vi "modbus slave new.vi"() -> ()   [LabVIEW 2016, in "MB SLAVE.lvlib"]
uses:
  MB SLAVE.lvlib
  <vilib>/NI/Modbus Library/Network Protocol/Network Slave/daemon status.ctl
  <vilib>/NI/Modbus Library/Network Protocol/Network Slave/TCP/Connection.ctl
  <vilib>/NI/Modbus Library/API/Wrapper/Create TCP Slave.vi
  <vilib>/NI/Modbus Library/API/slave/Modbus Slave.lvclass
  <vilib>/NI/Modbus Library/API/Wrapper/API Main.lvlib
  <vilib>/ptbypt/NI_PtbyPt.lvlib
  <vilib>/NI/Modbus Library/Network Protocol/Network Slave/Network Slave.lvclass
  <vilib>/NI/Modbus Library/Network Protocol/Network Slave/TCP/TCP Slave.lvclass
panel:
  in  "写入采配水关键参数":u16[](array[numeric])
  in  "写入校准点信息":u16[](array[numeric])
  in  "写入关键参数":u16[](array[numeric])
  in  "写入各参数测量间隔":u16[](array[numeric])
  out "读取各参数测量间隔":u16[](array[numeric])
  in  "写入试剂余量":u16[](array[numeric])
  out "TCP Connection List":T1[](array[typedef])
  out "TCP Connection Count":u32
  out "Daemon Status":T2
  out "读取关键参数":u16[](array[numeric])
  out "status":bool
  in  "写入系统仪器状态":u16[](array[numeric])
  out "读取反控命令":u16[](array[numeric])
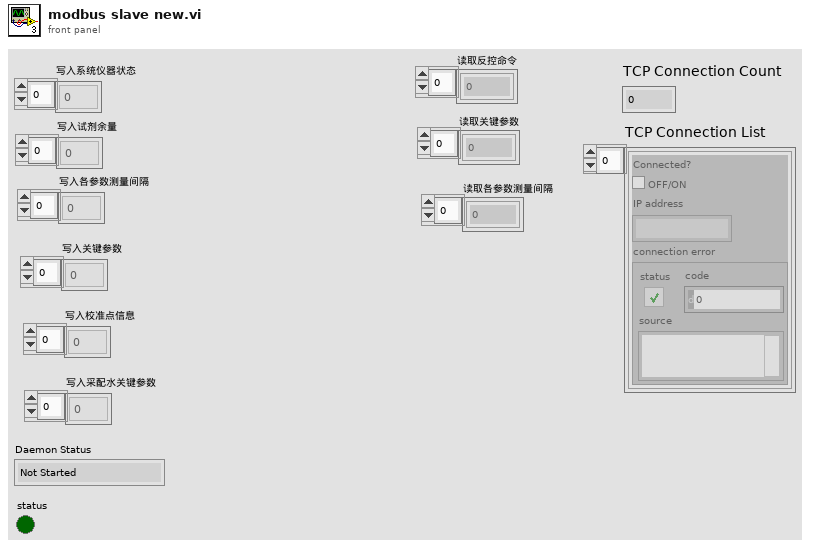
[diagram p1: front panel]
types:
  T1 = typedef "TCP Slave.lvclass/Connection.ctl" = cluster{"Connected?":bool, "IP address":string, "connection error":errorcluster}
  T2 = typedef "Network Slave.lvclass/daemon status.ctl" = enum16{"Not Started", "Running", "Error", "Stopped"}
  T3 = typedef "系统交互.ctl" = cluster{"运行模式":enum16{"维护模式", "常规模式", "应急模式", "质控模式", "性能测试"}, "运行间隔":i16, "流程运行中":bool, "自动运行启动参数":T4, "SYSTEM Interface.总磷总氮类型":enum16{"单模块", "总磷总氮二合一模块", "氨氮总磷二合一模块"}, "多参数运行间隔":i16, "配水时间":dbl, "沉淀时间":dbl, "清洗时间":dbl, "关键参数改变":bool, "温度告警":bool, "湿度告警":bool, "烟感告警":bool, "水浸告警":bool, "开门告警":bool, "SystemTask":enum16{"停机", "待机", "调试", "水样采集", "沉沙", "进样", "仪表测试分析", "反吹", "清洗", "除藻"}, "PumpState":enum16{"--", "只用泵1", "只用泵2", "双泵交替"}, "除藻选择":enum16{"不开除藻", "开除藻"}, "报警信息":enum16{"无报警", "断电报警", "采样管理欠压（源水泵故障）", "进样管路欠压（进样泵/增加泵故障）"}, "软件升级":bool}
  T4 = typedef "启动参数.ctl" = cluster{"氨氮":bool, "总磷":bool, "总氮":bool, "多参数":bool, "CODmn":bool, "CODCr":bool, "氟化物":bool, "超标留样":bool, "重金属":bool, "挥发酚":bool}
  T5 = typedef "多参数交互.ctl" = cluster{"pH":bool, "DO":bool, "Turb":bool, "Cond":bool, "Temp":bool, "叶绿素a启用":bool, "蓝绿藻":bool, "藻密度":bool, "orp":bool}
  T6 = typedef "CODMn交互.ctl" = cluster{"COD浓度（mg/L)":dbl, "水样启动时间":timestamp, "加标回收启动时间":timestamp, "CODMn工作状态":enum16{"空闲", "水样测试", "标样核查", "零点核查", "跨度核查", "空白测试", "平行样测试", "加标回收", "空白校准", "标样校准", "初始化（清洗）"}, "多列列表框":i32, "平台试剂余量百分比":sgl, "关键参数":cluster{"测量量程":dbl, "测量精度":dbl, "测量间隔":dbl, "消解温度":dbl, "消解时长":dbl, "空白校准时间":timestamp, "曲线截距":dbl, "曲线斜率":dbl, "测量检出限":dbl, "测量信号值":dbl, "线性相关系数":dbl, "二次多项式系数":dbl, "标样校准时间":timestamp, "稀释倍数":dbl, "三项式系数":dbl, "空白标定系数":dbl, "量程系数":dbl, "F0/ORPA":dbl, "F1/ORPB":dbl, "F2/ORPK":dbl, "F3":dbl, "F4":dbl, "F5":dbl, "F6":dbl, "F7":dbl, "X0/滴定数":dbl, "量程":dbl}, "关键参数改变":bool, "校准信息":cluster{"低标液1浓度":dbl, "低标液1信号值":dbl, "低标液1启用":u16, "低标液2浓度":dbl, "低标液2信号值":dbl, "低标液2启用":u16, "低标液3浓度":dbl, "低标液3信号值":dbl, "低标液3启用":u16, "低标液4浓度":dbl, "低标液4信号值":dbl, "低标液4启用":u16, "低标液5浓度":dbl, "低标液5信号值":dbl, "低标液5启用":u16, "高标液1浓度":dbl, "高标液1信号值":dbl, "高标液1启用":u16, "高标液2浓度":dbl, "高标液2信号值":dbl, "高标液2启用":u16, "高标液3浓度":dbl, "高标液3信号值":dbl, "高标液3启用":u16, "高标液4浓度":dbl, "高标液4信号值":dbl, "高标液4启用":u16, "高标液5浓度":dbl, "高标液5信号值":dbl, "高标液5启用":u16, "低斜率":dbl, "低截距":dbl, "低二次多项式系数":dbl, "低线性相关系数":dbl, "高斜率":dbl, "高截距":dbl, "高二次多项式系数":dbl, "高线性相关系数":dbl}, "校准信息改变":bool}
  T7 = typedef "CODCr交互.ctl" = cluster{"状态告警区":cluster{"系统时间":timestamp, "工作状态":u16, "测量模式":enum16{"待机", "连续模式", "周期模式", "定点模式", "受控模式", "手动模式"}, "告警代码":u16, "故障代码":u16, "日志代码":u16, "软件版本":u16, "F0":sgl, "F1":sgl, "F2":sgl, "F3":sgl, "T":sgl, "H":sgl, "id":u16, "flowid":u16, "量程":u16, "总磷控温温度1":sgl, "营养盐控温温度2":sgl, "ADC":sgl}, "平台试剂余量百分比":sgl, "关键参数":cluster{"测量量程":dbl, "测量精度":dbl, "测量间隔":dbl, "消解温度":dbl, "消解时长":dbl, "空白校准时间":timestamp, "曲线截距":dbl, "曲线斜率":dbl, "测量检出限":dbl, "测量信号值":dbl, "线性相关系数":dbl, "二次多项式系数":dbl, "标样校准时间":timestamp, "稀释倍数":dbl, "三项式系数":dbl, "空白标定系数":dbl, "量程系数":dbl, "F0/ORPA":dbl, "F1/ORPB":dbl, "F2/ORPK":dbl, "F3":dbl, "F4":dbl, "F5":dbl, "F6":dbl, "F7":dbl, "X0/滴定数":dbl, "量程":dbl}, "关键参数改变":bool, "校准信息":cluster{"低标液1浓度":dbl, "低标液1信号值":dbl, "低标液1启用":u16, "低标液2浓度":dbl, "低标液2信号值":dbl, "低标液2启用":u16, "低标液3浓度":dbl, "低标液3信号值":dbl, "低标液3启用":u16, "低标液4浓度":dbl, "低标液4信号值":dbl, "低标液4启用":u16, "低标液5浓度":dbl, "低标液5信号值":dbl, "低标液5启用":u16, "高标液1浓度":dbl, "高标液1信号值":dbl, "高标液1启用":u16, "高标液2浓度":dbl, "高标液2信号值":dbl, "高标液2启用":u16, "高标液3浓度":dbl, "高标液3信号值":dbl, "高标液3启用":u16, "高标液4浓度":dbl, "高标液4信号值":dbl, "高标液4启用":u16, "高标液5浓度":dbl, "高标液5信号值":dbl, "高标液5启用":u16, "低斜率":dbl, "低截距":dbl, "低二次多项式系数":dbl, "低线性相关系数":dbl, "高斜率":dbl, "高截距":dbl, "高二次多项式系数":dbl, "高线性相关系数":dbl}, "校准信息改变":bool}
  T8 = typedef "氨氮交互.ctl" = cluster{"状态告警区":cluster{"系统时间":timestamp, "工作状态":u16, "测量模式":enum16{"待机", "连续模式", "周期模式", "定点模式", "受控模式", "手动模式"}, "告警代码":u16, "故障代码":u16, "日志代码":u16, "软件版本":u16, "F0":sgl, "F1":sgl, "F2":sgl, "F3":sgl, "T":sgl, "H":sgl, "id":u16, "flowid":u16, "量程":u16, "总磷控温温度1":sgl, "营养盐控温温度2":sgl, "ADC":sgl}, "平台试剂余量百分比":sgl, "关键参数":cluster{"测量量程":dbl, "测量精度":dbl, "测量间隔":dbl, "消解温度":dbl, "消解时长":dbl, "空白校准时间":timestamp, "曲线截距":dbl, "曲线斜率":dbl, "测量检出限":dbl, "测量信号值":dbl, "线性相关系数":dbl, "二次多项式系数":dbl, "标样校准时间":timestamp, "稀释倍数":dbl, "三项式系数":dbl, "空白标定系数":dbl, "量程系数":dbl, "F0/ORPA":dbl, "F1/ORPB":dbl, "F2/ORPK":dbl, "F3":dbl, "F4":dbl, "F5":dbl, "F6":dbl, "F7":dbl, "X0/滴定数":dbl, "量程":dbl}, "关键参数改变":bool, "校准信息":cluster{"低标液1浓度":dbl, "低标液1信号值":dbl, "低标液1启用":u16, "低标液2浓度":dbl, "低标液2信号值":dbl, "低标液2启用":u16, "低标液3浓度":dbl, "低标液3信号值":dbl, "低标液3启用":u16, "低标液4浓度":dbl, "低标液4信号值":dbl, "低标液4启用":u16, "低标液5浓度":dbl, "低标液5信号值":dbl, "低标液5启用":u16, "高标液1浓度":dbl, "高标液1信号值":dbl, "高标液1启用":u16, "高标液2浓度":dbl, "高标液2信号值":dbl, "高标液2启用":u16, "高标液3浓度":dbl, "高标液3信号值":dbl, "高标液3启用":u16, "高标液4浓度":dbl, "高标液4信号值":dbl, "高标液4启用":u16, "高标液5浓度":dbl, "高标液5信号值":dbl, "高标液5启用":u16, "低斜率":dbl, "低截距":dbl, "低二次多项式系数":dbl, "低线性相关系数":dbl, "高斜率":dbl, "高截距":dbl, "高二次多项式系数":dbl, "高线性相关系数":dbl}, "校准信息改变":bool}
  T9 = typedef "总磷交互.ctl" = cluster{"状态告警区":cluster{"系统时间":timestamp, "工作状态":u16, "测量模式":enum16{"待机", "连续模式", "周期模式", "定点模式", "受控模式", "手动模式"}, "告警代码":u16, "故障代码":u16, "日志代码":u16, "软件版本":u16, "F0":sgl, "F1":sgl, "F2":sgl, "F3":sgl, "T":sgl, "H":sgl, "id":u16, "flowid":u16, "量程":u16, "总磷控温温度1":sgl, "营养盐控温温度2":sgl, "ADC":sgl}, "平台试剂余量百分比":sgl, "关键参数":cluster{"测量量程":dbl, "测量精度":dbl, "测量间隔":dbl, "消解温度":dbl, "消解时长":dbl, "空白校准时间":timestamp, "曲线截距":dbl, "曲线斜率":dbl, "测量检出限":dbl, "测量信号值":dbl, "线性相关系数":dbl, "二次多项式系数":dbl, "标样校准时间":timestamp, "稀释倍数":dbl, "三项式系数":dbl, "空白标定系数":dbl, "量程系数":dbl, "F0/ORPA":dbl, "F1/ORPB":dbl, "F2/ORPK":dbl, "F3":dbl, "F4":dbl, "F5":dbl, "F6":dbl, "F7":dbl, "X0/滴定数":dbl, "量程":dbl}, "关键参数改变":bool, "校准信息":cluster{"低标液1浓度":dbl, "低标液1信号值":dbl, "低标液1启用":u16, "低标液2浓度":dbl, "低标液2信号值":dbl, "低标液2启用":u16, "低标液3浓度":dbl, "低标液3信号值":dbl, "低标液3启用":u16, "低标液4浓度":dbl, "低标液4信号值":dbl, "低标液4启用":u16, "低标液5浓度":dbl, "低标液5信号值":dbl, "低标液5启用":u16, "高标液1浓度":dbl, "高标液1信号值":dbl, "高标液1启用":u16, "高标液2浓度":dbl, "高标液2信号值":dbl, "高标液2启用":u16, "高标液3浓度":dbl, "高标液3信号值":dbl, "高标液3启用":u16, "高标液4浓度":dbl, "高标液4信号值":dbl, "高标液4启用":u16, "高标液5浓度":dbl, "高标液5信号值":dbl, "高标液5启用":u16, "低斜率":dbl, "低截距":dbl, "低二次多项式系数":dbl, "低线性相关系数":dbl, "高斜率":dbl, "高截距":dbl, "高二次多项式系数":dbl, "高线性相关系数":dbl}, "校准信息改变":bool}
  T10 = typedef "总氮交互.ctl" = cluster{"状态告警区":cluster{"系统时间":timestamp, "工作状态":u16, "测量模式":enum16{"待机", "连续模式", "周期模式", "定点模式", "受控模式", "手动模式"}, "告警代码":u16, "故障代码":u16, "日志代码":u16, "软件版本":u16, "F0":sgl, "F1":sgl, "F2":sgl, "F3":sgl, "T":sgl, "H":sgl, "id":u16, "flowid":u16, "量程":u16, "总磷控温温度1":sgl, "营养盐控温温度2":sgl, "ADC":sgl}, "平台试剂余量百分比":sgl, "关键参数":cluster{"测量量程":dbl, "测量精度":dbl, "测量间隔":dbl, "消解温度":dbl, "消解时长":dbl, "空白校准时间":timestamp, "曲线截距":dbl, "曲线斜率":dbl, "测量检出限":dbl, "测量信号值":dbl, "线性相关系数":dbl, "二次多项式系数":dbl, "标样校准时间":timestamp, "稀释倍数":dbl, "三项式系数":dbl, "空白标定系数":dbl, "量程系数":dbl, "F0/ORPA":dbl, "F1/ORPB":dbl, "F2/ORPK":dbl, "F3":dbl, "F4":dbl, "F5":dbl, "F6":dbl, "F7":dbl, "X0/滴定数":dbl, "量程":dbl}, "关键参数改变":bool, "校准信息":cluster{"低标液1浓度":dbl, "低标液1信号值":dbl, "低标液1启用":u16, "低标液2浓度":dbl, "低标液2信号值":dbl, "低标液2启用":u16, "低标液3浓度":dbl, "低标液3信号值":dbl, "低标液3启用":u16, "低标液4浓度":dbl, "低标液4信号值":dbl, "低标液4启用":u16, "低标液5浓度":dbl, "低标液5信号值":dbl, "低标液5启用":u16, "高标液1浓度":dbl, "高标液1信号值":dbl, "高标液1启用":u16, "高标液2浓度":dbl, "高标液2信号值":dbl, "高标液2启用":u16, "高标液3浓度":dbl, "高标液3信号值":dbl, "高标液3启用":u16, "高标液4浓度":dbl, "高标液4信号值":dbl, "高标液4启用":u16, "高标液5浓度":dbl, "高标液5信号值":dbl, "高标液5启用":u16, "低斜率":dbl, "低截距":dbl, "低二次多项式系数":dbl, "低线性相关系数":dbl, "高斜率":dbl, "高截距":dbl, "高二次多项式系数":dbl, "高线性相关系数":dbl}, "校准信息改变":bool}
  T11 = cluster{"测量量程":dbl, "测量精度":dbl, "测量间隔":dbl, "消解温度":dbl, "消解时长":dbl, "空白校准时间":timestamp, "曲线截距":dbl, "曲线斜率":dbl, "测量检出限":dbl, "测量信号值":dbl, "线性相关系数":dbl, "二次多项式系数":dbl, "标样校准时间":timestamp, "稀释倍数":dbl, "三项式系数":dbl, "空白标定系数":dbl, "量程系数":dbl, "F0/ORPA":dbl, "F1/ORPB":dbl, "F2/ORPK":dbl, "F3":dbl, "F4":dbl, "F5":dbl, "F6":dbl, "F7":dbl, "X0/滴定数":dbl, "量程":dbl}
  T12 = cluster{"低标液1浓度":dbl, "低标液1信号值":dbl, "低标液1启用":u16, "低标液2浓度":dbl, "低标液2信号值":dbl, "低标液2启用":u16, "低标液3浓度":dbl, "低标液3信号值":dbl, "低标液3启用":u16, "低标液4浓度":dbl, "低标液4信号值":dbl, "低标液4启用":u16, "低标液5浓度":dbl, "低标液5信号值":dbl, "低标液5启用":u16, "高标液1浓度":dbl, "高标液1信号值":dbl, "高标液1启用":u16, "高标液2浓度":dbl, "高标液2信号值":dbl, "高标液2启用":u16, "高标液3浓度":dbl, "高标液3信号值":dbl, "高标液3启用":u16, "高标液4浓度":dbl, "高标液4信号值":dbl, "高标液4启用":u16, "高标液5浓度":dbl, "高标液5信号值":dbl, "高标液5启用":u16, "低斜率":dbl, "低截距":dbl, "低二次多项式系数":dbl, "低线性相关系数":dbl, "高斜率":dbl, "高截距":dbl, "高二次多项式系数":dbl, "高线性相关系数":dbl}
  T13 = enum16{"空闲", "水样测试", "标样核查", "零点核查", "跨度核查", "空白测试", "平行样测试", "加标回收", "空白校准", "标样校准", "初始化（清洗）"}
  T14 = typedef "超标留样交互.ctl" = cluster{"当前瓶号":u16}
  T15 = cluster{"测量量程":dbl, "测量精度":dbl, "测量间隔":dbl, "消解温度":dbl, "消解时长":dbl, "空白校准时间":timestamp, "曲线截距":dbl, "曲线斜率":dbl, "测量检出限":dbl, "测量信号值":dbl, "线性相关系数":dbl, "二次多项式系数":dbl, "标样校准时间":timestamp, "稀释倍数":dbl, "三项式系数":dbl, "空白标定系数":dbl, "量程系数":dbl, "F0/ORPA":dbl, "F1/ORPB":dbl, "F2/ORPK":dbl, "F3":dbl, "F4":dbl, "F5":dbl, "F6":dbl, "F7":dbl, "X0/滴定数":dbl, "量程":dbl}[]
  T16 = cluster{"低标液1浓度":dbl, "低标液1信号值":dbl, "低标液1启用":u16, "低标液2浓度":dbl, "低标液2信号值":dbl, "低标液2启用":u16, "低标液3浓度":dbl, "低标液3信号值":dbl, "低标液3启用":u16, "低标液4浓度":dbl, "低标液4信号值":dbl, "低标液4启用":u16, "低标液5浓度":dbl, "低标液5信号值":dbl, "低标液5启用":u16, "高标液1浓度":dbl, "高标液1信号值":dbl, "高标液1启用":u16, "高标液2浓度":dbl, "高标液2信号值":dbl, "高标液2启用":u16, "高标液3浓度":dbl, "高标液3信号值":dbl, "高标液3启用":u16, "高标液4浓度":dbl, "高标液4信号值":dbl, "高标液4启用":u16, "高标液5浓度":dbl, "高标液5信号值":dbl, "高标液5启用":u16, "低斜率":dbl, "低截距":dbl, "低二次多项式系数":dbl, "低线性相关系数":dbl, "高斜率":dbl, "高截距":dbl, "高二次多项式系数":dbl, "高线性相关系数":dbl}[]
  T17 = enum16{"启动整机", "停止整机", "标样核查", "加标回收", "平行样测试", "零点核查", "跨度核查", "校零", "校标"}
  T18 = cluster{"status":bool, "代码":u16, "source":string}
  T19 = enum16{"", "CODMn", "PH", "氨氮", "总氮", "总磷", "CODCr", "电导率", "水温", "溶解氧", "浊度", "叶绿素", "藻密度", "ORP"}
  T20 = enum16{"i13001", "i13002", "i13003", "i13004", "i13005", "i13006", "i13007", "i13008", "i13009", "i13010", "i13011", "i13012", "i13013", "i13014", "i13015", "i13016", "i13017", "i13101", "i13102", "i13103", "i13104", "i13105", "i13106", "i13107", "i13108", "i13109", "i13110"}
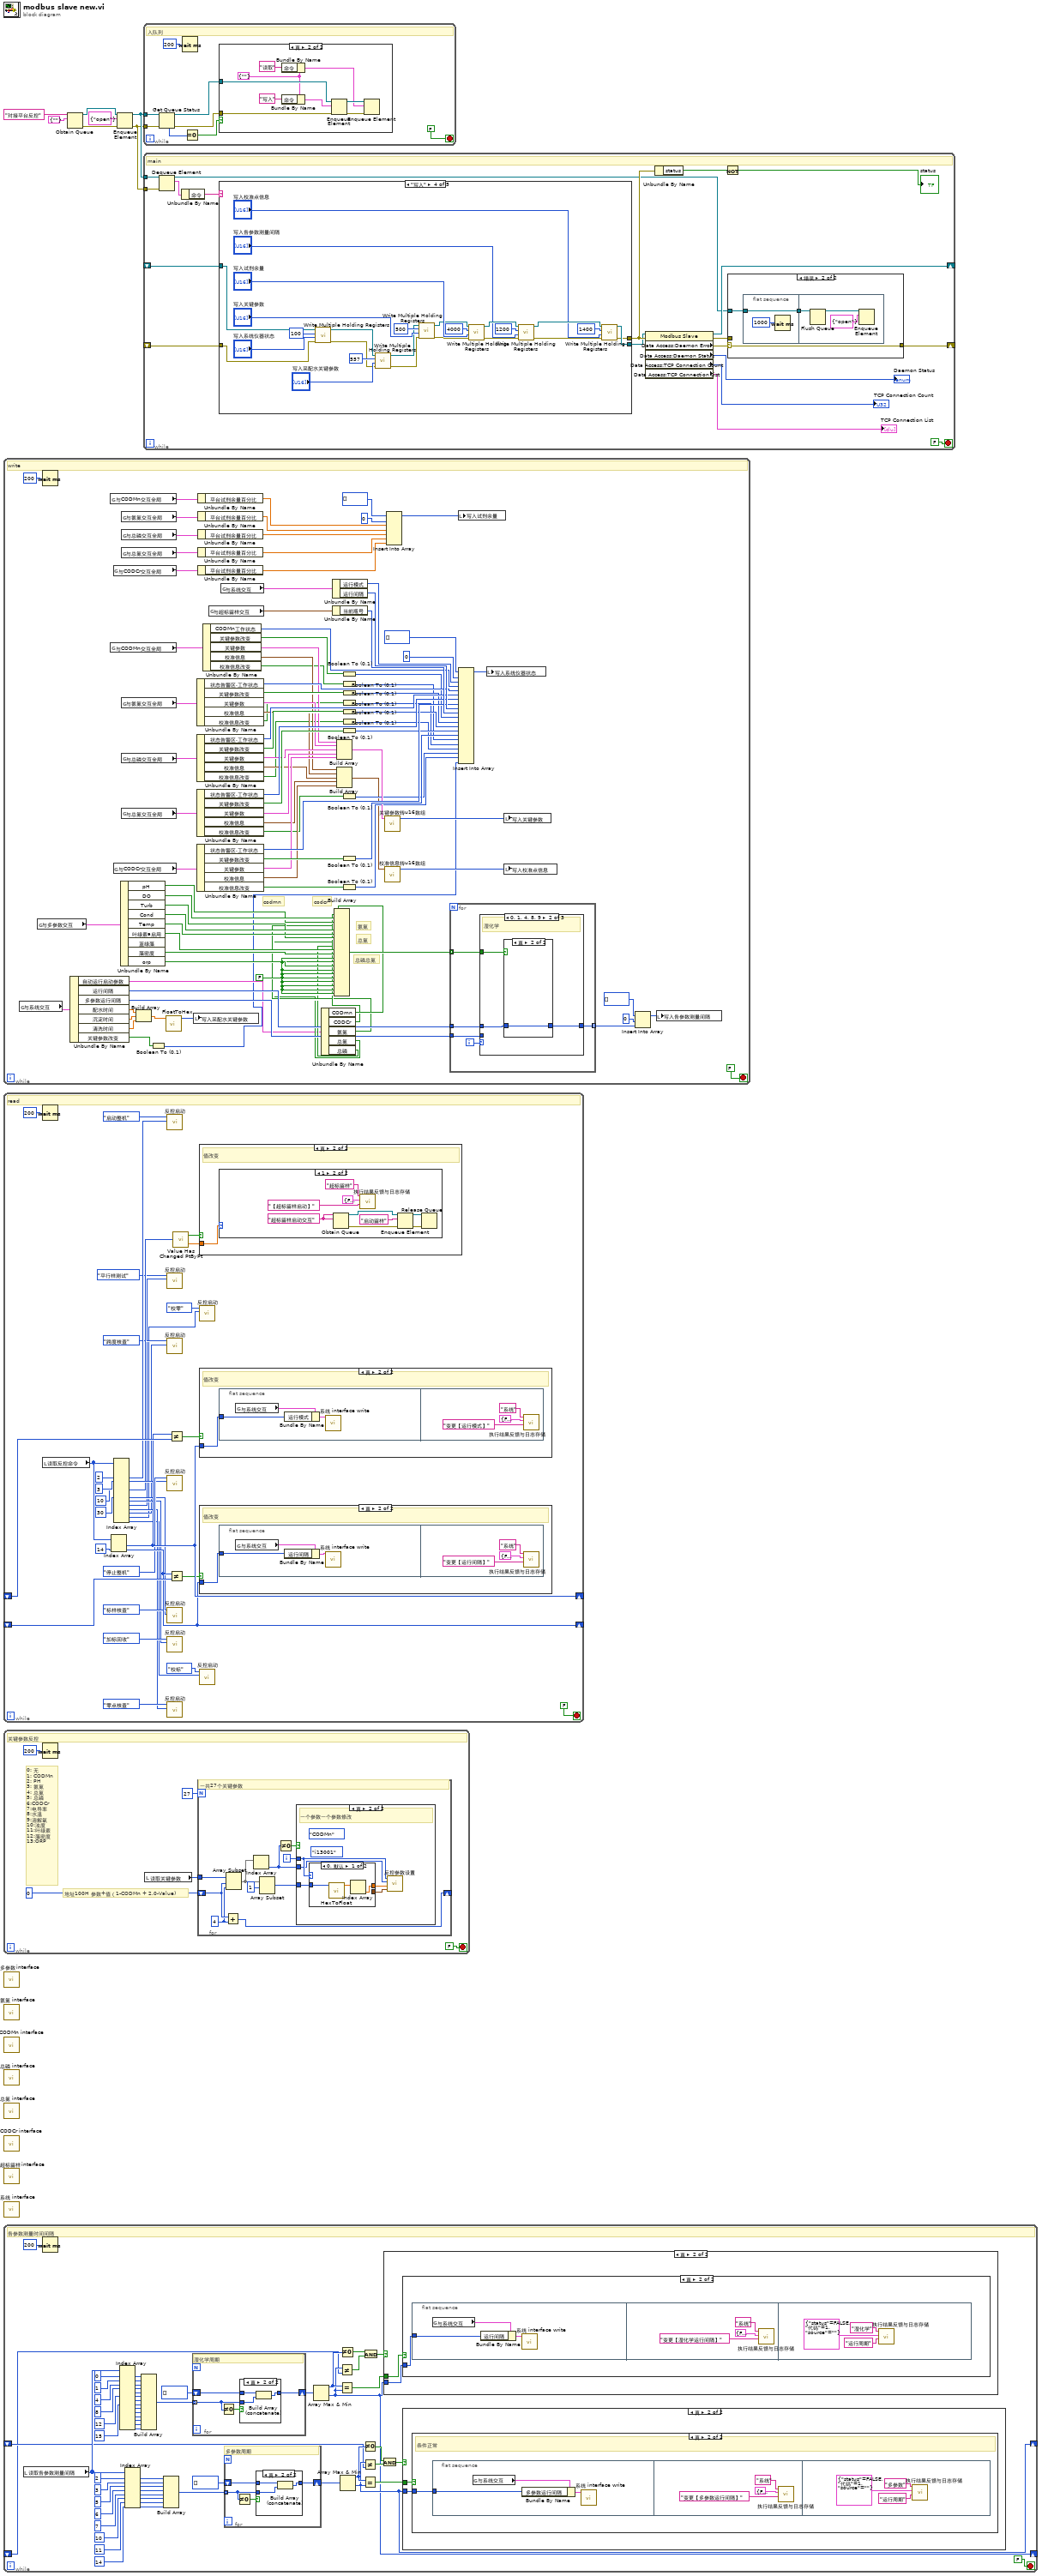
[diagram p0: block diagram]
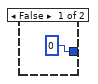
[diagram p3: hidden frame]
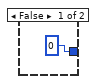
[diagram p4: hidden frame]
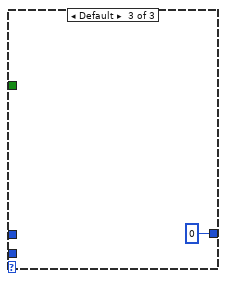
[diagram p5: hidden frame]
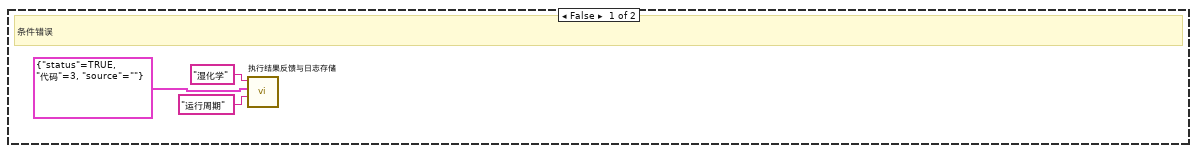
[diagram p7: hidden frame]
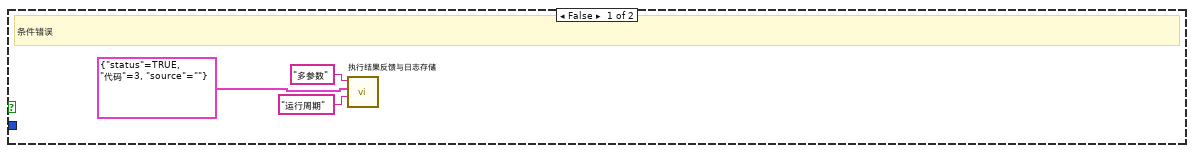
[diagram p9: hidden frame]
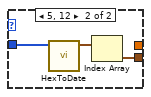
[diagram p13: hidden frame]
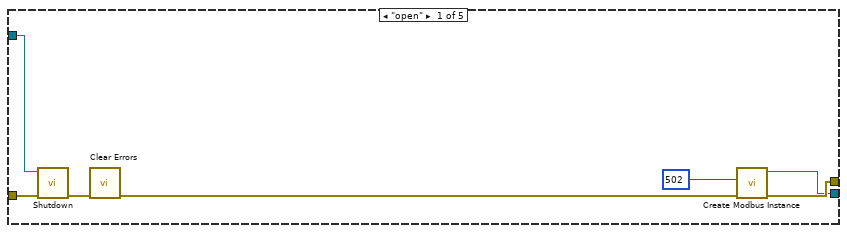
[diagram p20: hidden frame]
diagram:
  n1 = while {
    stop <- FALSE stop-if-true
    w59 = FALSE ("元素")
    # "总磷总氮"
    # "总氮"
    # "氨氮"
    # "codcr"
    # "codmn"
    # "write"
    n2 = global read "modbus slave全局.vi" "与系统交互"() -> (w72:T3)
    n3 = global read "modbus slave全局.vi" "与多参数交互"() -> (w71:T5)
    n4 = Wait (ms)(milliseconds to wait=u32 200 ("等待时间（毫秒）")) -> ()  [unwired: 1 out]
    n5 = Unbundle By Name(w72) -> ("自动运行启动参数"=w15:T4, "运行间隔"=w57:i16, "多参数运行间隔"=w56:i16, "配水时间"=w14:dbl, "沉淀时间"=w13:dbl, "清洗时间"=w12:dbl, "关键参数改变"=w9:bool)
    n6 = global read "modbus slave全局.vi" "与CODMn交互全局"() -> (w82:T6)
    n7 = global read "modbus slave全局.vi" "与CODMn交互全局"() -> (w90:T6)
    n8 = global read "modbus slave全局.vi" "与CODCr交互全局"() -> (w78:T7)
    n9 = global read "modbus slave全局.vi" "与CODCr交互全局"() -> (w98:T7)
    n10 = Unbundle By Name(w71) -> ("pH"=w66:bool, "DO"=w67:bool, "Turb"=w63:bool, "Cond"=w65:bool, "Temp"=w64:bool, "叶绿素a启用"=w62:bool, "藻密度"=w61:bool, "orp"=w60:bool)  [unwired: 1 out]
    n11 = global read "modbus slave全局.vi" "与氨氮交互全局"() -> (w81:T8)
    n12 = global read "modbus slave全局.vi" "与总磷交互全局"() -> (w80:T9)
    n13 = global read "modbus slave全局.vi" "与总氮交互全局"() -> (w79:T10)
    n14 = global read "modbus slave全局.vi" "与氨氮交互全局"() -> (w92:T8)
    n15 = global read "modbus slave全局.vi" "与总磷交互全局"() -> (w94:T9)
    n16 = global read "modbus slave全局.vi" "与总氮交互全局"() -> (w96:T10)
    n17 = Build Array(w14, w13, w12) -> (w11:dbl[])
    n18 = Boolean To (0,1)(Boolean=w9) -> (0, 1=w8:i16)
    n19 = call "FloatToHex.vi"("FLOAT"=w11) -> ("交织的数组"=w10:u16[])  [unwired: 10 in]
    n20 = local write "写入采配水关键参数"(w10) -> ()
    n21 = Unbundle By Name(w92) -> ("状态告警区.工作状态"=w93:u16, "关键参数改变"=w48:bool, "关键参数"=w43:T11, "校准信息"=w36:T12, "校准信息改变"=w30:bool)
    n22 = Unbundle By Name(w94) -> ("状态告警区.工作状态"=w95:u16, "关键参数改变"=w47:bool, "关键参数"=w42:T11, "校准信息"=w35:T12, "校准信息改变"=w28:bool)
    n23 = Unbundle By Name(w96) -> ("状态告警区.工作状态"=w97:u16, "关键参数改变"=w46:bool, "关键参数"=w41:T11, "校准信息"=w34:T12, "校准信息改变"=w26:bool)
    n24 = Unbundle By Name(w98) -> ("状态告警区.工作状态"=w99:u16, "关键参数改变"=w45:bool, "关键参数"=w40:T11, "校准信息"=w33:T12, "校准信息改变"=w24:bool)
    n25 = Unbundle By Name(w82) -> ("平台试剂余量百分比"=w77:sgl)
    n26 = Unbundle By Name(w81) -> ("平台试剂余量百分比"=w76:sgl)
    n27 = Unbundle By Name(w80) -> ("平台试剂余量百分比"=w75:sgl)
    n28 = Unbundle By Name(w79) -> ("平台试剂余量百分比"=w74:sgl)
    n29 = Unbundle By Name(w78) -> ("平台试剂余量百分比"=w73:sgl)
    n30 = Unbundle By Name(w90) -> ("CODMn工作状态"=w91:T13, "关键参数改变"=w49:bool, "关键参数"=w44:T11, "校准信息"=w37:T12, "校准信息改变"=w32:bool)
    n31 = global read "modbus slave全局.vi" "与超标留样交互"() -> (w103:T14)
    n32 = global read "modbus slave全局.vi" "与系统交互"() -> (w100:T3)
    n33 = Unbundle By Name(w15) -> ("CODmn"=w20:bool, "CODCr"=w19:bool, "氨氮"=w18:bool, "总氮"=w17:bool, "总磷"=w16:bool)
    n34 = Unbundle By Name(w100) -> ("运行模式"=w101:enum16{"维护模式", "常规模式", "应急模式", "质控模式", "性能测试"}, "运行间隔"=w102:i16)
    n35 = Unbundle By Name(w103) -> ("当前瓶号"=w104:u16)
    n36 = Build Array(w20, w19, w67, w66, w18, w65, w64, w63, w17, w16, w62, w61, w59, w59, w60, w59, w59, w59, w59, w59, w59, w59) -> (w58:bool[])
    n37 = Build Array(w44, w43, w42, w41, w40) -> (w39:T15)
    n38 = Build Array(w37, w36, w35, w34, w33) -> (w22:T16)
    n39 = Boolean To (0,1)(Boolean=w49) -> (0, 1=w54:i16)
    n40 = Boolean To (0,1)(Boolean=w32) -> (0, 1=w31:i16)
    n41 = Boolean To (0,1)(Boolean=w48) -> (0, 1=w53:i16)
    n42 = Boolean To (0,1)(Boolean=w30) -> (0, 1=w29:i16)
    n43 = Boolean To (0,1)(Boolean=w47) -> (0, 1=w52:i16)
    n44 = Boolean To (0,1)(Boolean=w28) -> (0, 1=w27:i16)
    n45 = Boolean To (0,1)(Boolean=w46) -> (0, 1=w51:i16)
    n46 = Boolean To (0,1)(Boolean=w26) -> (0, 1=w25:i16)
    n47 = Boolean To (0,1)(Boolean=w45) -> (0, 1=w50:i16)
    n48 = Boolean To (0,1)(Boolean=w24) -> (0, 1=w23:i16)
    n49 = call "关键参数转u16数组.vi"("关键参数"=w39) -> ("添加的数组"=w38:u16[])  [unwired: 10 in]
    n50 = call "校准信息转u16数组.vi"("关键参数"=w22) -> ("添加的数组"=w21:u16[])  [unwired: 10 in]
    n51 = Insert Into Array(array=u16[] [] ("values to write"), index=0 ("索引"), new element #1=w77, new element #2=w76, new element #3=w75, new element #4=w74, new element #5=w73) -> (w85:u16[])
    n52 = for {
      tunnel: w58 -> [w110] mode=indexing
      tunnel: w57 -> [w107]
      tunnel: w56 -> [w108]
      tunnel: [w106] -> w55 mode=indexing
      i -> [w109]
      n53 = case shown="0, 1, 4, 8, 9" w109 {
        tunnel: w110 -> [w112 w118 _]
        tunnel: w108 -> [w113 _ _]
        tunnel: w107 -> [_ w117 _]
        tunnel: [w111 w116 i16 0 ("运行间隔")] -> w106
        frame 2, 3, 5..7, 10, 11, 14 {
          # "多参数"
          n54 = case shown="真" w112 {
            tunnel: w113 -> [_ w115]
            tunnel: [i16 0 ("运行间隔") w115] -> w111
            frame False {
            }
            frame True {
            }
          }
        }
        frame 0, 1, 4, 8, 9 {
          # "湿化学"
          n55 = case shown="真" w118 {
            tunnel: w117 -> [_ w120]
            tunnel: [i16 0 ("运行间隔") w120] -> w116
            frame False {
            }
            frame True {
            }
          }
        }
        frame Default {
        }
      }
    }
    n56 = local write "写入试剂余量"(w85) -> ()
    n57 = Insert Into Array(array=u16[] [] ("values to write"), index=0 ("索引"), new element #1=w101, new element #2=w91, new element #3=w93, new element #4=w95, new element #5=w97, new element #6=w99, new element #7=w102, new element #8=w104, new element #9=w54, new element #10=w53, new element #11=w52, new element #12=w51, new element #13=w50, new element #14=w31, new element #15=w29, new element #16=w27, new element #17=w25, new element #18=w23, new element #19=w8) -> (w89:u16[])
    n58 = local write "写入系统仪器状态"(w89) -> ()
    n59 = local write "写入关键参数"(w38) -> ()
    n60 = local write "写入校准点信息"(w21) -> ()
    n61 = Insert Into Array(array=u16[] [] ("values to write"), index=0 ("索引"), new element=w55) -> (w68:u16[])
    n62 = local write "写入各参数测量间隔"(w68) -> ()
  }
  n63 = while {
    shift-right: [w151] -> _
    shift-left: _ -> [w153]
    shift-right: [w148] -> _
    shift-left: _ -> [w150]
    stop <- FALSE stop-if-true
    # "read"
    n64 = Wait (ms)(milliseconds to wait=u32 200 ("等待时间（毫秒）")) -> ()  [unwired: 1 out]
    n65 = local read "读取反控命令"() -> (w143:u16[])
    n66 = Index Array(array=w143, index #2=14 ("索引")) -> (element #1=w151:u16, element #2=w148:u16)  [unwired: 1 in]
    n67 = Index Array(array=w143, index #3=2 ("索引"), index #4=3 ("索引"), index #6=10 ("索引"), index #8=30 ("索引")) -> (element #3=w142:u16, element #4=w139:u16, element #6=w136:u16, element #8=w134:u16, element #9=w128:u16, element #10=w127:u16, element #11=w126:u16, element #12=w124:u16, element #13=w123:u16, element #14=w122:u16)  [unwired: 10 in, 4 out]
    n68 = call "反控启动.vi"("启动参数"=w142, "启动类型"=T17."启动整机") -> ()  [unwired: 10 in]
    n69 = call "反控启动.vi"("启动参数"=w127, "启动类型"=T17."平行样测试") -> ()  [unwired: 10 in]
    n70 = call "反控启动.vi"("启动参数"=w124, "启动类型"=T17."跨度核查") -> ()  [unwired: 10 in]
    n71 = call "反控启动.vi"("启动参数"=w139, "启动类型"=T17."停止整机") -> ()  [unwired: 10 in]
    n72 = call "反控启动.vi"("启动参数"=w134, "启动类型"=T17."标样核查") -> ()  [unwired: 10 in]
    n73 = call "反控启动.vi"("启动参数"=w128, "启动类型"=T17."加标回收") -> ()  [unwired: 10 in]
    n74 = call "反控启动.vi"("启动参数"=w126, "启动类型"=T17."零点核查") -> ()  [unwired: 10 in]
    n75 = Not Equal?(x=w151, y=w153) -> (x != y?=w152:bool)
    n76 = Not Equal?(x=w148, y=w150) -> (x != y?=w149:bool)
    n77 = call <vilib>:"Value Has Changed PtByPt.vi"("input data point"=w136) -> ("has changed"=w138:bool, "output data point"=w137:dbl)  [unwired: 1 in]
    n78 = case shown="真" w138 {
      tunnel: w137 -> [_ w157]
      frame False {
      }
      frame True {
        # "值改变"
        n79 = case shown="1" w157 {
          frame 0, Default {
          }
          frame 1 {
            w162 = "超标留样启动交互" ("名称（未命名）")
            n80 = Obtain Queue(name (unnamed)=w162, element data type=w162) -> (queue out=w158:refnum<queue>, error out=w159:errorcluster)  [unwired: 3 in, 1 out]
            n81 = call "执行结果反馈与日志存储.vi"("日志信息"="【超标留样启动】", "error out"=T18 {"status"=FALSE, "代码"=1, "source"=""}, "设备"="超标留样") -> ()  [unwired: 9 in]
            n82 = Enqueue Element(queue=w158, element="启动留样" ("名称（未命名）"), error in (no error)=w159) -> (queue out=w160:refnum<queue>, error out=w161:errorcluster)  [unwired: 1 in, 1 out]
            n83 = Release Queue(queue=w160, error in (no error)=w161) -> ()  [unwired: 1 in, 3 out]
          }
        }
      }
    }
    n84 = call "反控启动.vi"("启动参数"=w123, "启动类型"=T17."校零") -> ()  [unwired: 10 in]
    n85 = case shown="真" w152 {
      tunnel: w151 -> [_ w174]
      frame False {
      }
      frame True {
        # "值改变"
        n86 = flat-sequence {
          tunnel: w174 -> [w175]
          frame #0 {
            n87 = global read "modbus slave全局.vi" "与系统交互"() -> (w177:T3)
            n88 = Bundle By Name(cluster=w177, "运行模式"=w175) -> (w176:T3)
            n89 = call "系统 interface write.vi"("与系统交互"=w176) -> ()  [unwired: 11 in]
          }
          frame #1 {
            n90 = call "执行结果反馈与日志存储.vi"("日志信息"="变更【运行模式】", "error out"=T18 {"status"=FALSE, "代码"=1, "source"=""}, "设备"="系统") -> ()  [unwired: 9 in]
          }
        }
      }
    }
    n91 = case shown="真" w149 {
      tunnel: w148 -> [_ w167]
      frame False {
      }
      frame True {
        # "值改变"
        n92 = flat-sequence {
          tunnel: w167 -> [w169]
          frame #0 {
            n93 = global read "modbus slave全局.vi" "与系统交互"() -> (w170:T3)
            n94 = Bundle By Name(cluster=w170, "运行间隔"=w169) -> (w168:T3)
            n95 = call "系统 interface write.vi"("与系统交互"=w168) -> ()  [unwired: 11 in]
          }
          frame #1 {
            n96 = call "执行结果反馈与日志存储.vi"("日志信息"="变更【运行间隔】", "error out"=T18 {"status"=FALSE, "代码"=1, "source"=""}, "设备"="系统") -> ()  [unwired: 9 in]
          }
        }
      }
    }
    n97 = call "反控启动.vi"("启动参数"=w122, "启动类型"=T17."校标") -> ()  [unwired: 10 in]
  }
  n98 = while {
    stop <- FALSE stop-if-true
    # "地址100H 参数+值（1-CODMn + 2.0-Value)"
    # "0: 无\n1: CODMn\n2: PH\n3: 氨氮\n4: 总氮\n5: 总磷\n6:CODCr\n7:电导率\n8:水温\n9:溶解氧\n10:浊度\n11:叶绿素\n12:藻密度\n13:ORP"
    # "关键参数反控"
    n99 = Wait (ms)(milliseconds to wait=u32 200 ("等待时间（毫秒）")) -> ()  [unwired: 1 out]
    n100 = local read "读取关键参数"() -> (w183:u16[])
    n101 = for {
      N: 27 -> [_]
      tunnel: w183 -> [w195]
      shift-right: [w186] -> _
      shift-left: 0 ("索引") -> [w188]
      i -> [w191]
      w187 = 4 ("长度")
      # "一共27个关键参数"
      n102 = Add(x=w188, y=w187) -> (x+y=w186:i32)
      n103 = Array Subset(array=w195, index=w188, length=w187) -> (w194:u16[])
      n104 = Index Array(array=w194) -> (element=w190:u16)  [unwired: 1 in]
      n105 = Array Subset(array=w194, index=1 ("索引")) -> (w192:u16[])  [unwired: 1 in]
      n106 = Not Equal To 0?(x=w190) -> (x != 0?=w189:bool)
      n107 = case shown="真" w189 {
        tunnel: w192 -> [_ w200]
        tunnel: w191 -> [_ w199]
        tunnel: w190 -> [_ w198]
        frame False {
        }
        frame True {
          (unwired) T19."CODMn"
          (unwired) T20."i13001" ("设置类型")
          # "一个参数一个参数修改"
          n108 = case shown="0, 默认" w199 {
            tunnel: w200 -> [w202 w205]
            tunnel: [_ w206] -> w196
            tunnel: [w203 _] -> w197
            frame 0, Default {
              n109 = call "HexToFloat.vi"("数组"=w202) -> ("FLOAT"=w201:sgl[])  [unwired: 10 in]
              n110 = Index Array(array=w201) -> (element=w203:sgl)  [unwired: 1 in]
            }
            frame 5, 12 {
              n111 = call "HexToDate.vi"("数组"=w205) -> ("DATE"=w204:timestamp[])  [unwired: 10 in]
              n112 = Index Array(array=w204) -> (element=w206:timestamp)  [unwired: 1 in]
            }
          }
          n113 = call "反控参数设置.vi"("value time"=w196, "value float"=w197, "设置参数"=w198, "设置类型"=w199) -> ()  [unwired: 8 in]
        }
      }
    }
  }
  n114 = call "多参数 interface.vi"() -> ()  [unwired: 12 in]
  n115 = call "氨氮 interface.vi"() -> ()  [unwired: 12 in]
  n116 = call "CODMn interface.vi"() -> ()  [unwired: 12 in]
  n117 = call "总磷 interface.vi"() -> ()  [unwired: 12 in]
  n118 = call "总氮 interface.vi"() -> ()  [unwired: 12 in]
  n119 = call "CODCr interface.vi"() -> ()  [unwired: 12 in]
  n120 = call "超标留样 interface.vi"() -> ()  [unwired: 12 in]
  n121 = call "系统 interface.vi"() -> ()  [unwired: 12 in]
  n122 = while {
    shift-right: [w218] -> _
    shift-left: _ -> [w217]
    shift-right: [w211] -> _
    shift-left: _ -> [w210]
    stop <- FALSE stop-if-true
    # "各参数测量时间间隔"
    n123 = local read "读取各参数测量间隔"() -> (w259:u16[])
    n124 = Wait (ms)(milliseconds to wait=u32 200 ("等待时间（毫秒）")) -> ()  [unwired: 1 out]
    n125 = Index Array(array=w259, index #1=0 ("索引"), index #2=1 ("索引"), index #3=4 ("索引"), index #4=8 ("索引"), index #6=12 ("索引"), index #8=15 ("索引")) -> (element #1=w240:u16, element #2=w239:u16, element #3=w238:u16, element #4=w237:u16, element #5=w236:u16, element #6=w235:u16, element #7=w234:u16, element #8=w233:u16, element #9=w232:u16, element #10=w231:u16, element #11=w230:u16, element #12=w229:u16, element #13=w228:u16, element #14=w227:u16)  [unwired: 8 in]
    n126 = Index Array(array=w259, index #1=2 ("索引"), index #2=3 ("索引"), index #3=5 ("索引"), index #4=6 ("索引"), index #5=7 ("索引"), index #6=10 ("索引"), index #7=11 ("索引"), index #8=14 ("索引")) -> (element #1=w248:u16, element #2=w247:u16, element #3=w246:u16, element #4=w245:u16, element #5=w244:u16, element #6=w243:u16, element #7=w242:u16, element #8=w241:u16)
    n127 = Build Array(w240, w239, w238, w237, w236, w235, w234, w233, w232, w231, w230, w229, w228, w227) -> (w222:u16[])
    n128 = Build Array(w248, w247, w246, w245, w244, w243, w242, w241) -> (w226:u16[])
    n129 = for {
      shift-right: [w297] -> w221
      shift-left: u16[] [] ("添加的数组") -> [w298]
      tunnel: w222 -> [w296] mode=indexing
      # "湿化学周期"
      n130 = Not Equal To 0?(x=w296) -> (x != 0?=w299:bool)
      n131 = case shown="真" w299 {
        tunnel: w298 -> [w300 w303]
        tunnel: w296 -> [_ w302]
        tunnel: [w300 w301] -> w297
        frame False {
        }
        frame True {
          n132 = Build Array (concatenate)(w303, w302) -> (w301:u16[])
        }
      }
    }
    n133 = for {
      tunnel: w226 -> [w306] mode=indexing
      shift-right: [w304] -> w224
      shift-left: u16[] [] ("添加的数组") -> [w307]
      # "多参数周期"
      n134 = Not Equal To 0?(x=w306) -> (x != 0?=w305:bool)
      n135 = case shown="真" w305 {
        tunnel: w307 -> [w308 w311]
        tunnel: w306 -> [_ w310]
        tunnel: [w308 w309] -> w304
        frame False {
        }
        frame True {
          n136 = Build Array (concatenate)(w311, w310) -> (w309:u16[])
        }
      }
    }
    n137 = Array Max & Min(array=w221) -> (max value=w220:u16, min value=w211:u16)  [unwired: 2 out]
    n138 = Not Equal?(x=w211, y=w210) -> (x != y?=w209:bool)
    n139 = Equal?(x=w220, y=w211) -> (x = y?=w207:bool)
    n140 = Not Equal To 0?(x=w220) -> (x != 0?=w212:bool)
    n141 = Array Max & Min(array=w224) -> (max value=w219:u16, min value=w218:u16)  [unwired: 2 out]
    n142 = Not Equal To 0?(x=w219) -> (x != 0?=w216:bool)
    n143 = Not Equal?(x=w218, y=w217) -> (x != y?=w215:bool)
    n144 = Equal?(x=w219, y=w218) -> (x = y?=w213:bool)
    n145 = And(x=w212, y=w209) -> (x .and. y?=w208:bool)
    n146 = And(x=w216, y=w215) -> (x .and. y?=w214:bool)
    n147 = case shown="真" w208 {
      tunnel: w211 -> [_ w267]
      tunnel: w207 -> [_ w266]
      frame False {
        # "值未改变"
      }
      frame True {
        n148 = case shown="真" w266 {
          tunnel: w267 -> [_ w271]
          frame False {
            # "条件错误"
            n149 = call "执行结果反馈与日志存储.vi"("日志信息"="运行周期", "error out"=T18 {"status"=TRUE, "代码"=3, "source"=""}, "设备"="湿化学") -> ()  [unwired: 9 in]
          }
          frame True {
            n150 = flat-sequence {
              tunnel: w271 -> [w273]
              frame #0 {
                n151 = global read "modbus slave全局.vi" "与系统交互"() -> (w274:T3)
                n152 = Bundle By Name(cluster=w274, "运行间隔"=w273) -> (w272:T3)
                n153 = call "系统 interface write.vi"("与系统交互"=w272) -> ()  [unwired: 11 in]
              }
              frame #1 {
                n154 = call "执行结果反馈与日志存储.vi"("日志信息"="变更【湿化学运行间隔】", "error out"=T18 {"status"=FALSE, "代码"=1, "source"=""}, "设备"="系统") -> ()  [unwired: 9 in]
              }
              frame #2 {
                n155 = call "执行结果反馈与日志存储.vi"("日志信息"="运行周期", "error out"=T18 {"status"=FALSE, "代码"=1, "source"=""}, "设备"="湿化学") -> ()  [unwired: 9 in]
              }
            }
          }
        }
      }
    }
    n156 = case shown="真" w214 {
      tunnel: w218 -> [_ w282]
      tunnel: w213 -> [_ w281]
      frame False {
        # "值未改变"
      }
      frame True {
        n157 = case shown="真" w281 {
          tunnel: w282 -> [_ w286]
          frame False {
            # "条件错误"
            n158 = call "执行结果反馈与日志存储.vi"("日志信息"="运行周期", "error out"=T18 {"status"=TRUE, "代码"=3, "source"=""}, "设备"="多参数") -> ()  [unwired: 9 in]
          }
          frame True {
            # "条件正常"
            n159 = flat-sequence {
              tunnel: w286 -> [w288]
              frame #0 {
                n160 = global read "modbus slave全局.vi" "与系统交互"() -> (w289:T3)
                n161 = Bundle By Name(cluster=w289, "多参数运行间隔"=w288) -> (w287:T3)
                n162 = call "系统 interface write.vi"("与系统交互"=w287) -> ()  [unwired: 11 in]
              }
              frame #1 {
                n163 = call "执行结果反馈与日志存储.vi"("日志信息"="变更【多参数运行间隔】", "error out"=T18 {"status"=FALSE, "代码"=1, "source"=""}, "设备"="系统") -> ()  [unwired: 9 in]
              }
              frame #2 {
                n164 = call "执行结果反馈与日志存储.vi"("日志信息"="运行周期", "error out"=T18 {"status"=FALSE, "代码"=1, "source"=""}, "设备"="多参数") -> ()  [unwired: 9 in]
              }
            }
          }
        }
      }
    }
  }
  n165 = Obtain Queue(name (unnamed)="对接平台反控" ("名称（未命名）"), element data type=cluster{"命令":string} {"命令"=""}) -> (queue out=w5:refnum<queue>, error out=w4:errorcluster)  [unwired: 3 in, 1 out]
  n166 = Enqueue Element(queue=w5, element=cluster{"命令":string} {"命令"="open"} ("元素"), error in (no error)=w4) -> (queue out=w2:refnum<queue>, error out=w1:errorcluster)  [unwired: 1 in, 1 out]
  n167 = while {
    tunnel: w2 -> [w319]
    tunnel: w1 -> [w317]
    stop <- FALSE stop-if-true
    # "入队列"
    n168 = Get Queue Status(queue=w319, error in (no error)=w317) -> (queue out=w318:refnum<queue>, error out=w316:errorcluster, # elements in queue=w315:i32)  [unwired: 1 in, 5 out]
    n169 = Wait (ms)(milliseconds to wait=u32 200 ("等待时间（毫秒）")) -> ()  [unwired: 1 out]
    n170 = Equal To 0?(x=w315) -> (x = 0?=w314:bool)
    n171 = case shown="真" w314 {
      tunnel: w318 -> [_ w328]
      tunnel: w316 -> [_ w327]
      frame False {
      }
      frame True {
        w323 = cluster{"命令":string} {"命令"=""} ("元素")
        n172 = Bundle By Name(cluster=w323, "命令"="读取") -> (w320:cluster{"命令":string})
        n173 = Bundle By Name(cluster=w323, "命令"="写入") -> (w322:cluster{"命令":string})
        n174 = Enqueue Element(queue=w328, element=w322, error in (no error)=w327) -> (queue out=w326:refnum<queue>, error out=w325:errorcluster)  [unwired: 1 in, 1 out]
        n175 = Enqueue Element(queue=w326, element=w320, error in (no error)=w325) -> ()  [unwired: 1 in, 3 out]
      }
    }
  }
  n176 = while {
    tunnel: w2 -> [w347]
    tunnel: w1 -> [w346]
    shift-right: [w336] -> _
    shift-left: _ -> [w343]
    shift-right: [w332] -> _
    shift-left: _ -> [w342]
    stop <- FALSE stop-if-true
    # "main"
    n177 = Dequeue Element(queue=w347, error in (no error)=w346) -> (queue out=w334:refnum<queue>, element=w345:cluster{"命令":string})  [unwired: 1 in, 2 out]
    n178 = Unbundle By Name(w345) -> ("命令"=w344:string)
    n179 = case shown="\"写入\"" w344 {
      tunnel: [w360 w363 w367 w395 w414] -> w337
      tunnel: [w361 w364 w366 w393 w413] -> w338
      tunnel: w343 -> [w359 w363 w382 w411 w416]
      tunnel: w342 -> [w358 w365 w381 w410 w415]
      frame "open" {
        n180 = call-dynamic "Shutdown.vi"("error in"=w358, "Modbus slave in"=w359) -> ("error out"=w357:errorcluster)  [unwired: 9 in]
        n181 = call <vilib>:"Clear Errors.vi"("error in (no error)"=w357) -> ("error out"=w356:errorcluster)  [unwired: 5 in, 1 out]
        n182 = call-poly <vilib>:"Create Modbus Instance.vi"("error in"=w356, "port (502)"=u16 502) -> ("error out"=w361:errorcluster, "TCP slave instance"=w360:refnum<class "Modbus Slave.lvclass">)  [unwired: 8 in]
      }
      frame "close" {
        n183 = call-dynamic "Shutdown.vi"("error in"=w365, "Modbus slave in"=w363) -> ("error out"=w364:errorcluster)  [unwired: 9 in]
      }
      frame "读取", Default {
        n184 = call-dynamic "Read Holding Registers.vi"("error in"=w381, "number of inputs"=u16 40, "starting address"=u16 0, "Modbus slave in"=w382) -> ("error out"=w373:errorcluster, "register values"=w378:u16[], "Modbus slave out"=w374:refnum<class "Modbus Slave.lvclass">)  [unwired: 5 in]
        n185 = case shown="无错误" w373 {
          tunnel: w378 -> [w385 _]
          frame No Error {
            "读取反控命令" <- w385
          }
          frame Error {
          }
        }
        n186 = call-dynamic "Read Holding Registers.vi"("error in"=w373, "number of inputs"=u16 256, "starting address"=u16 256, "Modbus slave in"=w374) -> ("error out"=w368:errorcluster, "register values"=w377:u16[], "Modbus slave out"=w369:refnum<class "Modbus Slave.lvclass">)  [unwired: 5 in]
        n187 = case shown="无错误" w368 {
          tunnel: w377 -> [w384 _]
          frame No Error {
            "读取关键参数" <- w384
          }
          frame Error {
          }
        }
        n188 = call-dynamic "Read Holding Registers.vi"("error in"=w368, "number of inputs"=u16 22, "starting address"=u16 1000, "Modbus slave in"=w369) -> ("error out"=w366:errorcluster, "register values"=w370:u16[], "Modbus slave out"=w367:refnum<class "Modbus Slave.lvclass">)  [unwired: 5 in]
        n189 = case shown="无错误" w366 {
          tunnel: w370 -> [w383 _]
          frame No Error {
            "读取各参数测量间隔" <- w383
          }
          frame Error {
          }
        }
      }
      frame "写入" {
        n190 = call-dynamic "Write Multiple Holding Registers.vi"("error in"=w410, "registers to write"="写入系统仪器状态", "starting address"=u16 100, "Modbus slave in"=w411) -> ("error out"=w387:errorcluster, "Modbus slave out"=w390:refnum<class "Modbus Slave.lvclass">)  [unwired: 6 in]
        n191 = call-dynamic "Write Multiple Holding Registers.vi"("error in"=w387, "registers to write"="写入采配水关键参数", "starting address"=u16 557, "Modbus slave in"=w390) -> ("error out"=w386:errorcluster, "Modbus slave out"=w389:refnum<class "Modbus Slave.lvclass">)  [unwired: 6 in]
        n192 = call-dynamic "Write Multiple Holding Registers.vi"("error in"=w386, "registers to write"="写入关键参数", "starting address"=u16 500, "Modbus slave in"=w389) -> ("error out"=w400:errorcluster, "Modbus slave out"=w401:refnum<class "Modbus Slave.lvclass">)  [unwired: 6 in]
        n193 = call-dynamic "Write Multiple Holding Registers.vi"("error in"=w400, "registers to write"="写入试剂余量", "starting address"=u16 4000, "Modbus slave in"=w401) -> ("error out"=w404:errorcluster, "Modbus slave out"=w405:refnum<class "Modbus Slave.lvclass">)  [unwired: 6 in]
        n194 = call-dynamic "Write Multiple Holding Registers.vi"("error in"=w404, "registers to write"="写入各参数测量间隔", "starting address"=u16 1200, "Modbus slave in"=w405) -> ("error out"=w394:errorcluster, "Modbus slave out"=w396:refnum<class "Modbus Slave.lvclass">)  [unwired: 6 in]
        n195 = call-dynamic "Write Multiple Holding Registers.vi"("error in"=w394, "registers to write"="写入校准点信息", "starting address"=u16 1400, "Modbus slave in"=w396) -> ("error out"=w393:errorcluster, "Modbus slave out"=w395:refnum<class "Modbus Slave.lvclass">)  [unwired: 6 in]
      }
      frame "反馈" {
        n196 = global read "modbus slave全局.vi" "执行结果反馈"() -> (w412:u16[])
        n197 = call-dynamic "Write Multiple Holding Registers.vi"("error in"=w415, "registers to write"=w412, "starting address"=u16 4608, "Modbus slave in"=w416) -> ("error out"=w413:errorcluster, "Modbus slave out"=w414:refnum<class "Modbus Slave.lvclass">)  [unwired: 6 in]
      }
    }
    n198 = property class="Modbus Slave"(reference=w337, error in=w338) -> (reference out=w336:refnum<class "Modbus Slave.lvclass">, error out=w333:errorcluster, "Data Access:Daemon Error"=w335:errorcluster, "Data Access:Daemon Status"=→"Daemon Status":T2, "Data Access:TCP Connection Count"=→"TCP Connection Count":u32, "Data Access:TCP Connection List"=→"TCP Connection List":T1[])
    n199 = Unbundle By Name(w338) -> ("status"=w340:bool)
    n200 = Not(x=w340) -> (.not. x?=→"status":bool)
    n201 = case shown="错误" w335 {
      selector: w335 -> [_ w348]
      tunnel: w334 -> [_ w350]
      tunnel: w333 -> [_ _]
      tunnel: [_ w348] -> w332
      frame No Error {
      }
      frame Error {
        n202 = flat-sequence {
          tunnel: w350 -> [w352]
          tunnel: [w352] -> w349
          tunnel: w349 -> [w355]
          frame #0 {
            n203 = Wait (ms)(milliseconds to wait=u32 1000 ("等待时间（毫秒）")) -> ()  [unwired: 1 out]
          }
          frame #1 {
            n204 = Flush Queue(queue=w355) -> (queue out=w353:refnum<queue>)  [unwired: 1 in, 2 out]
            n205 = Enqueue Element(queue=w353, element=cluster{"命令":string} {"命令"="open"} ("元素")) -> ()  [unwired: 2 in, 3 out]
          }
        }
      }
    }
  }
